vi "Merge Error Wire.vi"(7 "Call Chain (F)":bool, 10 "MultiErrors in":refnum<class "MultiErrors.lvclass">, 11 "error in (no error)":errorcluster) -> (2 "MultiErrors out":refnum<class "MultiErrors.lvclass">)   [LabVIEW 2020, in "Volatus.lvlib" / "MultiErrors.lvclass"]
uses:
  MultiErrors.lvclass
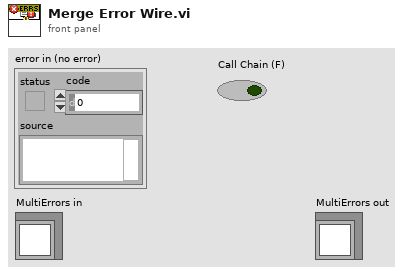
[diagram p1: front panel]
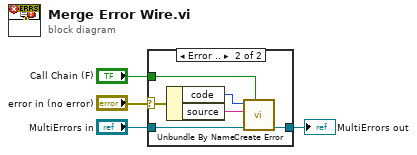
[diagram p0: block diagram]
diagram:
  n1 = case shown="Error .." "error in (no error)" {
    selector: "error in (no error)" -> [_ w10]
    tunnel: "MultiErrors in" -> [w5 w7]
    tunnel: "Call Chain (F)" -> [_ w11]
    tunnel: [w5 w6] -> w1
    frame No Error {
    }
    frame Error {
      n2 = Unbundle By Name(w10) -> ("code"=w8:i32, "source"=w9:string)
      n3 = call "Create Error.vi"("Call Chain (F)"=w11, "MultiErrors in"=w7, "Message"=w9, "Code"=w8) -> ("MultiErrors out"=w6:refnum<class "MultiErrors.lvclass">)  [unwired: 7 in]
    }
  }
  "MultiErrors out" <- w1
